vi "InitialPermutation.vi"(0 "Numeric":u64 format="%064b") -> (1 "Right":bool[](array[boolean]), 2 "Left":bool[](array[boolean]))   [LabVIEW 2013]
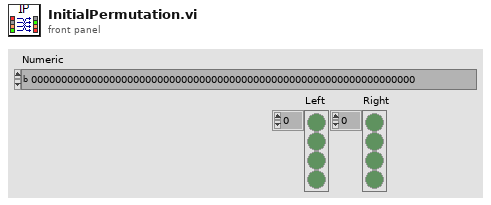
[diagram p1: front panel]
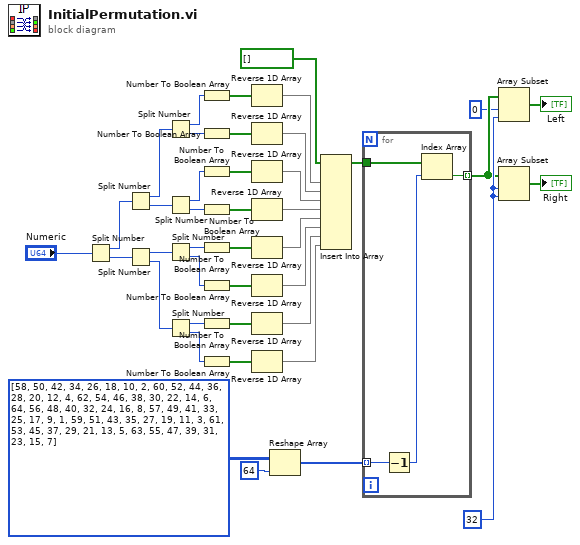
[diagram p0: block diagram]
diagram:
  w22 = 32 ("length")
  n1 = Split Number(x="Numeric") -> (hi(x)=w40:u32, lo(x)=w35:u32)
  n2 = Split Number(x=w40) -> (hi(x)=w39:u16, lo(x)=w38:u16)
  n3 = Split Number(x=w35) -> (hi(x)=w36:u16, lo(x)=w37:u16)
  n4 = Split Number(x=w39) -> (hi(x)=w34:u8, lo(x)=w33:u8)
  n5 = Split Number(x=w38) -> (hi(x)=w32:u8, lo(x)=w31:u8)
  n6 = Split Number(x=w36) -> (hi(x)=w30:u8, lo(x)=w29:u8)
  n7 = Split Number(x=w37) -> (hi(x)=w28:u8, lo(x)=w27:u8)
  n8 = Number To Boolean Array(number=w34) -> (Boolean array=w21:bool[])
  n9 = Number To Boolean Array(number=w33) -> (Boolean array=w19:bool[])
  n10 = Number To Boolean Array(number=w32) -> (Boolean array=w17:bool[])
  n11 = Number To Boolean Array(number=w31) -> (Boolean array=w15:bool[])
  n12 = Number To Boolean Array(number=w30) -> (Boolean array=w13:bool[])
  n13 = Number To Boolean Array(number=w29) -> (Boolean array=w11:bool[])
  n14 = Number To Boolean Array(number=w28) -> (Boolean array=w9:bool[])
  n15 = Number To Boolean Array(number=w27) -> (Boolean array=w7:bool[])
  n16 = Reverse 1D Array(array=w21) -> (reversed array=w20:bool[])
  n17 = Reverse 1D Array(array=w19) -> (reversed array=w18:bool[])
  n18 = Reverse 1D Array(array=w17) -> (reversed array=w16:bool[])
  n19 = Reverse 1D Array(array=w15) -> (reversed array=w14:bool[])
  n20 = Reverse 1D Array(array=w13) -> (reversed array=w12:bool[])
  n21 = Reverse 1D Array(array=w11) -> (reversed array=w10:bool[])
  n22 = Reverse 1D Array(array=w9) -> (reversed array=w8:bool[])
  n23 = Reverse 1D Array(array=w7) -> (reversed array=w6:bool[])
  n24 = Reshape Array(u8[][] [[58, 50, 42, 34, 26, 18, 10, 2], [60, 52, 44, 36, 28, 20, 12, 4], [62, 54, 46, 38, 30, 22, 14, 6], [64, 56, 48, 40, 32, 24, 16, 8], [57, 49, 41, 33, 25, 17, 9, 1], [59, 51, 43, 35, 27, 19, 11, 3], [61, 53, 45, 37, 29, 21, 13, 5], [63, 55, 47, 39, 31, 23, 15, 7]], 64 ("dimension size")) -> (w24:u8[])
  n25 = Insert Into Array(array=bool[] [], new element #1=w20, new element #2=w18, new element #3=w16, new element #4=w14, new element #5=w12, new element #6=w10, new element #7=w8, new element #8=w6) -> (w3:bool[])  [unwired: 1 in]
  n26 = for {
    tunnel: w3 -> [w44]
    tunnel: w24 -> [w45] mode=indexing
    tunnel: [w42] -> w2 mode=indexing
    n27 = Decrement(x=w45) -> (x-1=w43:u8)
    n28 = Index Array(array=w44, index=w43) -> (element=w42:bool)
  }
  n29 = Array Subset(array=w2, index=0, length=w22) -> (→"Left":bool[])
  n30 = Array Subset(array=w2, index=w22, length=w22) -> (→"Right":bool[])
